vi "GetRemoteControl.vi"(0 "reference in":refnum<class "Button.lvclass">, 11 "Error In":errorcluster) -> (4 "reference out":refnum<class "Button.lvclass">, 8 "RemoteControl":refnum<class "RemoteControl.lvclass">, 15 "Error Out":errorcluster)   [LabVIEW 2024, in "Button.lvclass"]
uses:
  Button.lvclass
  RemoteControl_class/RemoteControl.lvclass
  Button.lvclass/Button.ctl
panel:
  # "Connector Pane"
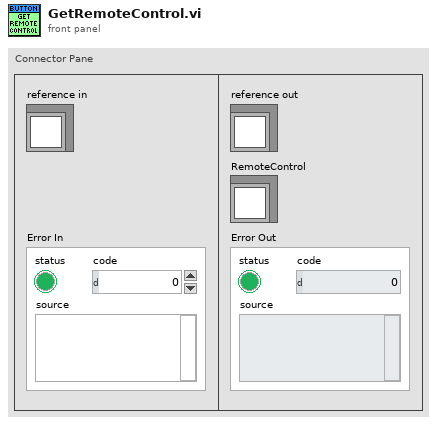
[diagram p1: front panel]
types:
  T1 = typedef "Button.lvclass/ObjectAttributes.ctl" = cluster{"RemoteControl":refnum<class "RemoteControl.lvclass">}
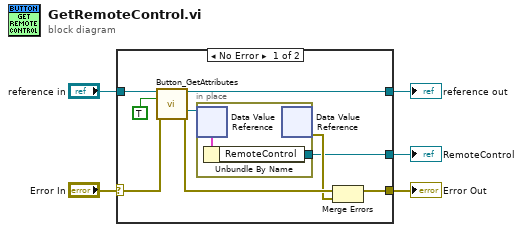
[diagram p0: block diagram]
diagram:
  n1 = case shown="No Error" "Error In" {
    selector: "Error In" -> [w14 w18]
    tunnel: [w12 w18] -> w4
    tunnel: [w9 w17] -> w2
    tunnel: "reference in" -> [w10 w17]
    tunnel: [w8 _] -> w1
    frame No Error {
      n2 = call "Button_GetAttributes.vi"("reference in"=w10, "OnlyGetDvrReference(False)"=TRUE, "Error In"=w14) -> ("reference out"=w9:refnum<class "Button.lvclass">, "DataRef"=w6:refnum<data-value>, "Error Out"=w13:errorcluster)  [unwired: 9 in, 1 out]
      n3 = in-place {
        in-place-border: [w16] -> w8
        n4 = in-place-dvr #1(w6) -> (w15:T1)  [unwired: 1 out]
        n5 = Unbundle By Name(w15) -> ("RemoteControl"=w16:refnum<class "RemoteControl.lvclass">)
        n6 = in-place-dvr #1() -> (w11:errorcluster)  [unwired: 1 in, 1 out]
      }
      n7 = Merge Errors(w13, w11) -> (w12:errorcluster)
    }
    frame Error {
    }
  }
  "Error Out" <- w4
  "reference out" <- w2
  "RemoteControl" <- w1
